vi "Test Write Speed.vi"(8 "error in (no error)":errorcluster, 11 "LVtoITX in":refnum<class "LVtoITX.lvclass">) -> (0 "error out":errorcluster, 3 "LVtoITX out":refnum<class "LVtoITX.lvclass">)   [LabVIEW 2016, in "LVtoITX.lvclass"]
uses:
  LVtoITX.lvclass
panel:
  out "Numeric 2":i32
  out "Numeric":i32
  in  "length":i32=250
  out "convert ITX to TDMS (ms/file)":u32
  out "convert ITX to HDF5 (ms/file)":u32
  in  "ITX Path":path
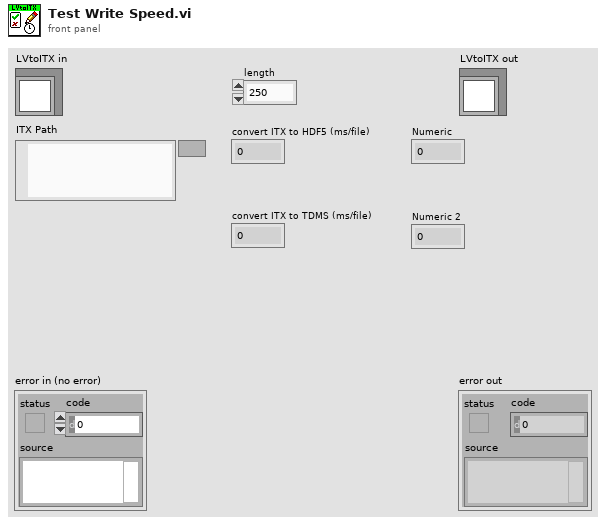
[diagram p1: front panel]
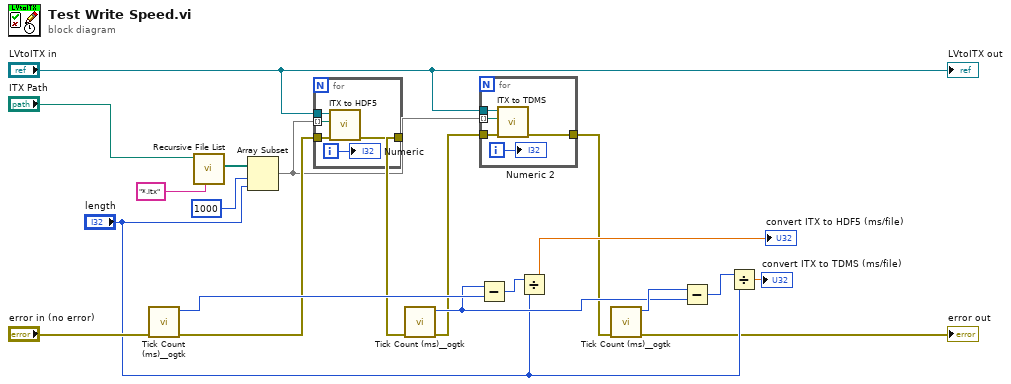
[diagram p0: block diagram]
diagram:
  n1 = call <userlib>:"Tick Count (ms)__ogtk.vi"("error in (no error)"="error in (no error)") -> ("error out"=w11:errorcluster, "millisecond timer value"=w18:u32)  [unwired: 9 in]
  n2 = call <vilib>:"Recursive File List.vi"("pattern"="*.itx", "Folder Path"="ITX Path") -> ("All Files in Dir"=w12:path[])  [unwired: 5 in, 4 out]
  n3 = Array Subset(array=w12, index=1000, length="length") -> (w9:path[])
  n4 = for {
    tunnel: "LVtoITX in" -> [w25]
    tunnel: w9 -> [w24] mode=indexing
    tunnel: w11 -> [w23]
    tunnel: [w22] -> w10
    i -> [w21]
    n5 = call "ITX to HDF5.vi"("error in (no error)"=w23, "file (use dialog)"=w24, "LVtoITX in"=w25) -> ("error out"=w22:errorcluster)  [unwired: 7 in, 1 out]
    "Numeric" <- w21
  }
  n6 = call <userlib>:"Tick Count (ms)__ogtk.vi"("error in (no error)"=w10) -> ("error out"=w7:errorcluster, "millisecond timer value"=w16:u32)  [unwired: 9 in]
  n7 = Subtract(x=w16, y=w18) -> (x-y=w15:u32)
  n8 = for {
    tunnel: w9 -> [w30] mode=indexing
    tunnel: "LVtoITX in" -> [w29]
    tunnel: w7 -> [w28]
    tunnel: [w27] -> w3
    i -> [w26]
    n9 = call "ITX to TDMS.vi"("error in (no error)"=w28, "file (use dialog)"=w30, "LVtoITX in"=w29) -> ("error out"=w27:errorcluster)  [unwired: 7 in, 1 out]
    "Numeric 2" <- w26
  }
  n10 = Divide(x=w15, y="length") -> (x/y=→"convert ITX to HDF5 (ms/file)":dbl)
  n11 = call <userlib>:"Tick Count (ms)__ogtk.vi"("error in (no error)"=w3) -> ("error out"=→"error out":errorcluster, "millisecond timer value"=w17:u32)  [unwired: 9 in]
  n12 = Subtract(x=w17, y=w16) -> (x-y=w6:u32)
  n13 = Divide(x=w6, y="length") -> (x/y=→"convert ITX to TDMS (ms/file)":dbl)
  "LVtoITX out" <- "LVtoITX in"
